vi "Read IOCardIndex.vi"(8 "error in (no error)":errorcluster, 11 "Station Action in":refnum<class "Station Action.lvclass">) -> (0 "error out":errorcluster, 2 "IOCardIndex":i32, 3 "Station Action out":refnum<class "Station Action.lvclass">)   [LabVIEW 2019, in "Station Action.lvclass"]
uses:
  Station Action.lvclass
  Station Action.lvclass/Station Action.ctl
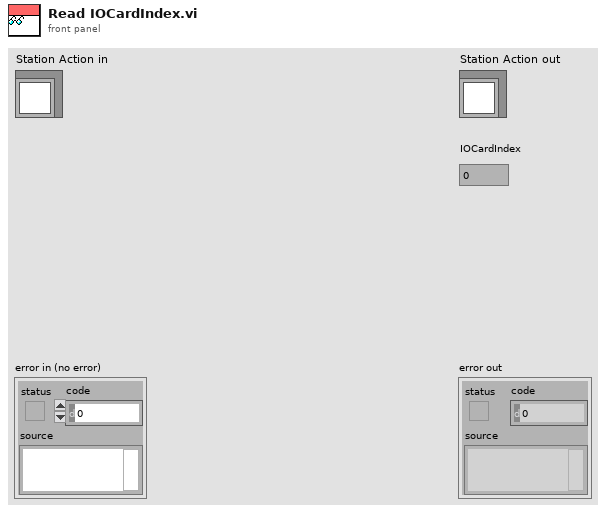
[diagram p1: front panel]
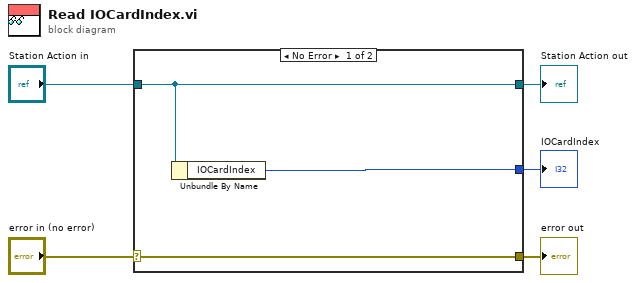
[diagram p0: block diagram]
diagram:
  n1 = case shown="No Error" "error in (no error)" {
    selector: "error in (no error)" -> [w8 w9]
    tunnel: [w8 w9] -> w4
    tunnel: [w7 w10] -> w2
    tunnel: "Station Action in" -> [w7 w10]
    tunnel: [w6 _] -> w1
    frame No Error {
      n2 = Unbundle By Name(w7) -> ("IOCardIndex"=w6:i32)
    }
    frame Error {
    }
  }
  "error out" <- w4
  "Station Action out" <- w2
  "IOCardIndex" <- w1
